vi "WFGenA01DC.vi"(1 "Param 0: Inactive":dbl, 2 "Param 1: Inactive":dbl, 3 "Param 2: Inactive":dbl, 4 "Param 3: Inactive":dbl, 5 "error in (no error)":errorcluster, 8 "WFParameters":T2={"Fs (Hz)"=20000.0, "Amp (V)"=5.0, "Ramp (s)"=0.005, "Dur (s)"=0.25} {"Dur (s)" min=0.0 format="%#_4g"; "Ramp (s)" min=0.0; "Fs (Hz)" min=0.0}, 10 "WFRepetitions":T1={"Del (s)"=0.0, "Int (s)"=0.0, "N"=1} {"Int (s)" min=0.0 format="%#_4g"; "Del (s)" min=0.0 format="%#_4f"}) -> (14 "Waveform Out":waveform(dbl), 19 "error out":errorcluster)   [LabVIEW 2013]
uses:
  util/impl/WFComposeA.vi
  WFParameters.ctl
  WFRepetitions.ctl
panel:
  out "Waveform Graph":waveform(dbl)(graph)
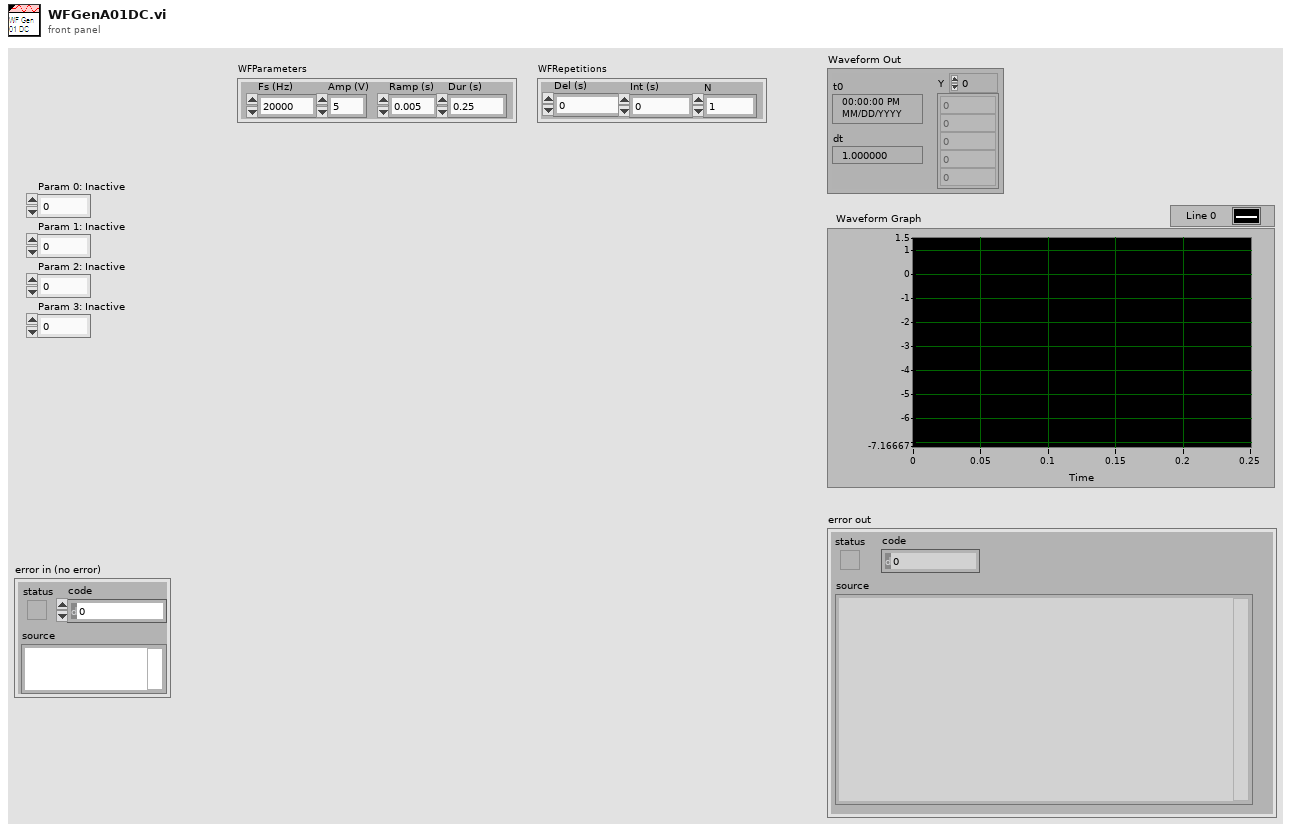
[diagram p1: front panel]
types:
  T1 = typedef "WFRepetitions.ctl" = cluster{"Del (s)":dbl, "Int (s)":dbl, "N":i32}
  T2 = typedef "WFParameters.ctl" = cluster{"Fs (Hz)":dbl, "Amp (V)":dbl, "Ramp (s)":dbl, "Dur (s)":dbl}
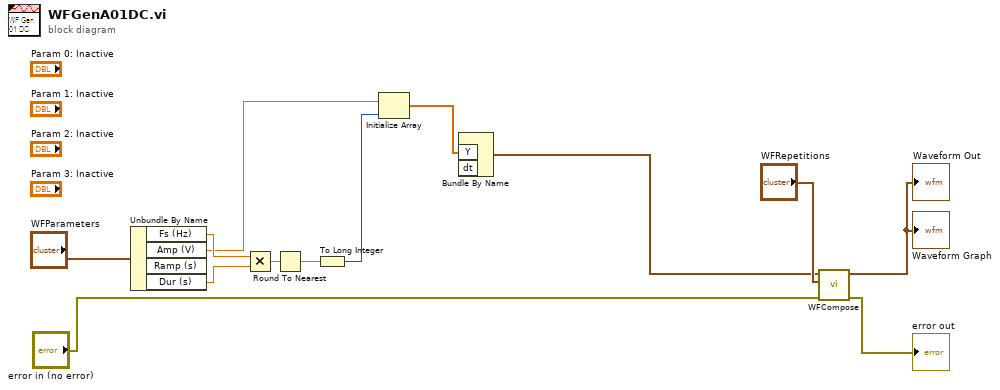
[diagram p0: block diagram]
diagram:
  n1 = Unbundle By Name("WFParameters") -> ("Fs (Hz)"=w9:dbl, "Amp (V)"=w7:dbl, "Dur (s)"=w10:dbl)  [unwired: 1 out]
  n2 = Multiply(x=w9, y=w10) -> (x*y=w2:dbl)
  n3 = Round To Nearest(number=w2) -> (nearest integer value=w1:dbl)
  n4 = To Long Integer(number=w1) -> (32bit integer=w8:i32)
  n5 = Initialize Array(w7, w8) -> (w6:dbl[])
  n6 = Bundle By Name("Y"=w6) -> (w5:waveform(dbl))  [unwired: 2 in]
  n7 = call-poly "WFCompose.vi"("error in (no error)"="error in (no error)", "WFRepetitions"="WFRepetitions", "Waveform In"=w5) -> ("error out"=→"error out":errorcluster, "Analog Waveform Out"=→"Waveform Graph" →"Waveform Out":waveform(dbl))  [unwired: 7 in]
